vi "LecturaPM.vi"() -> ()   [LabVIEW 2014]
panel:
  in  "Comando":string
  out "Respuesta Power Meter":string
  in  "Puerto":refnum<visa-resource-name>
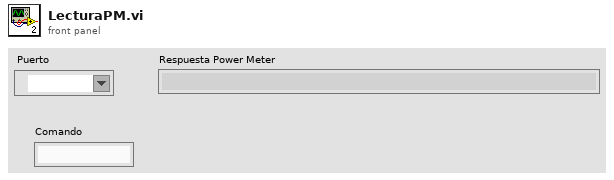
[diagram p1: front panel]
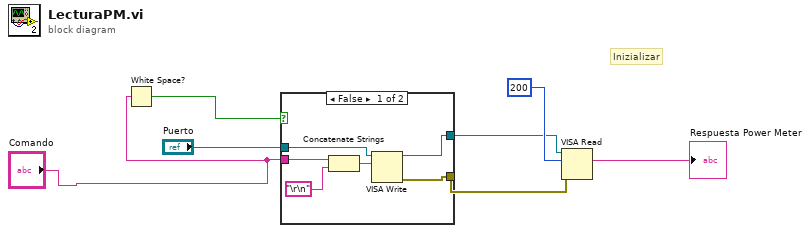
[diagram p0: block diagram]
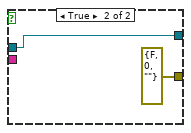
[diagram p2: hidden frame]
diagram:
  # "Inizializar"
  n1 = White Space?(1:"Comando") -> (0:w6:bool)
  n2 = case shown="False" w6 {
    tunnel: "Puerto" -> [w11 w15]
    tunnel: [w10 w15] -> w4
    tunnel: "Comando" -> [w9 _]
    tunnel: [w8 errorcluster {"status"=FALSE, "code"=0, "source"=""} ("error out")] -> w3
    frame False {
      n3 = Concatenate Strings(w9, "\r\n") -> (w12:string)
      n4 = VISA Write(VISA resource name=w11, write buffer=w12) -> (VISA resource name out=w10:refnum<visa-resource-name>, error out=w8:errorcluster)  [unwired: 1 in, 1 out]
    }
    frame True {
    }
  }
  n5 = VISA Read(VISA resource name=w4, byte count=u32 200 ("Byte Count (0)"), error in (no error)=w3) -> (read buffer=→"Respuesta Power Meter":string)  [unwired: 3 out]
